vi "mergeScriptEventLists.vi"(8 "error in (no error)":errorcluster, 10 "Array":refnum<class "ScriptEventList.lvclass">[](array[class]), 11 "ScriptEventList in":refnum<class "ScriptEventList.lvclass">) -> (0 "error out":errorcluster, 3 "ScriptEventList out":refnum<class "ScriptEventList.lvclass">)   [LabVIEW 2011, in "Tools.lvlib" / "Scripting.lvlib" / "ScriptEventList.lvclass"]
uses:
  ScriptEventList.lvclass
  ScriptEventList.lvclass/ScriptEventList.ctl
  ScriptEvent.lvclass
panel:
  out "Array 2":dbl[](array[numeric])
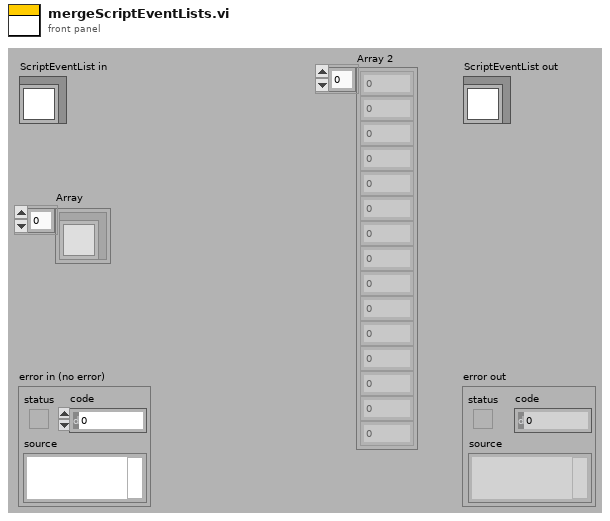
[diagram p1: front panel]
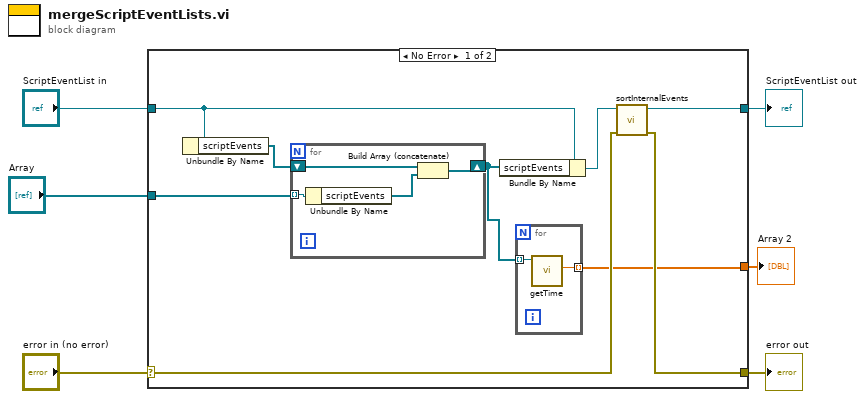
[diagram p0: block diagram]
diagram:
  n1 = case shown="No Error" "error in (no error)" {
    selector: "error in (no error)" -> [w11 w23]
    tunnel: [w9 w23] -> w5
    tunnel: [w10 w22] -> w3
    tunnel: "ScriptEventList in" -> [w13 w22]
    tunnel: "Array" -> [w15 _]
    tunnel: [w7 _] -> w1
    frame No Error {
      n2 = Unbundle By Name(w13) -> ("scriptEvents"=w14:refnum<class "ScriptEvent.lvclass">[])
      n3 = for {
        tunnel: w15 -> [w21] mode=indexing
        shift-right: [w19] -> w8
        shift-left: w14 -> [w20]
        n4 = Unbundle By Name(w21) -> ("scriptEvents"=w18:refnum<class "ScriptEvent.lvclass">[])
        n5 = Build Array (concatenate)(w20, w18) -> (w19:refnum<class "ScriptEvent.lvclass">[])
      }
      n6 = Bundle By Name(cluster=w13, "scriptEvents"=w8) -> (w12:refnum<class "ScriptEventList.lvclass">)
      n7 = for {
        tunnel: w8 -> [w17] mode=indexing
        tunnel: [w16] -> w7 mode=indexing
        n8 = call "getTime.vi"("ScriptEvent.lvclass in"=w17) -> ("time"=w16:dbl)  [unwired: 8 in, 2 out]
      }
      n9 = call "sortInternalEvents.vi"("error in (no error)"=w11, "ScriptEventList in"=w12) -> ("error out"=w9:errorcluster, "ScriptEventList out"=w10:refnum<class "ScriptEventList.lvclass">)  [unwired: 8 in]
    }
    frame Error {
    }
  }
  "error out" <- w5
  "ScriptEventList out" <- w3
  "Array 2" <- w1
